vi "Read.vi"(8 "error in (no error)":errorcluster, 9 "Timeout (ms)":i32, 10 "Bytes to Read":i32, 11 "TCP Connection in":refnum<class "TCP Connection.lvclass">) -> (0 "error out":errorcluster, 1 "TimeOut?":bool, 2 "Data":string, 3 "TCP Connection out":refnum<class "TCP Connection.lvclass">)   [LabVIEW 2020, in "TCP Connection.lvclass"]
uses:
  <vilib>/gpm_packages/@cs/Network-interface/Source/TCP Interface/TCP Connection/TCP Connection.lvclass
  <vilib>/gpm_packages/@cs/Network-interface/Source/TCP Interface/TCP Connection/TCP Connection.lvclass/TCP Connection.ctl
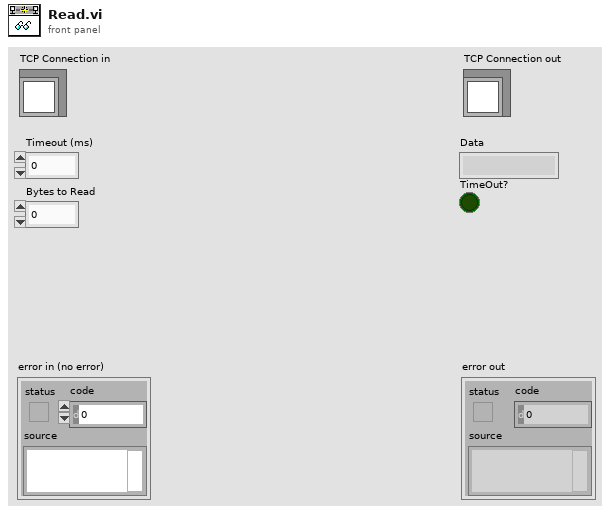
[diagram p1: front panel]
types:
  T1 = enum16{"Standard", "Buffered", "CRLF", "Immediate"}
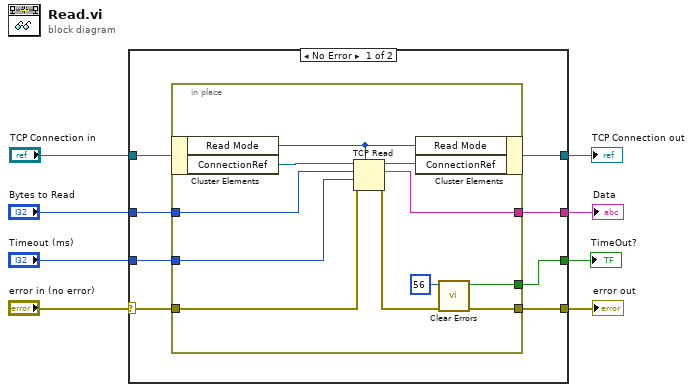
[diagram p0: block diagram]
diagram:
  n1 = case shown="No Error" "error in (no error)" {
    selector: "error in (no error)" -> [w15 w28]
    tunnel: "TCP Connection in" -> [w16 w29]
    tunnel: "Timeout (ms)" -> [w14 _]
    tunnel: "Bytes to Read" -> [w13 _]
    tunnel: [w12 w28] -> w4
    tunnel: [w11 _] -> w3
    tunnel: [w10 _] -> w2
    tunnel: [w9 w29] -> w1
    frame No Error {
      n2 = in-place {
        in-place-border: w15 -> [w25]
        in-place-border: w14 -> [w24]
        in-place-border: w13 -> [w23]
        in-place-border: [w21] -> w12
        in-place-border: [w19] -> w11
        in-place-border: [w18] -> w10
        n3 = in-place-cluster #1(w16) -> ("Read Mode"=w17:T1, "ConnectionRef"=w27:refnum<k5>)
        n4 = TCP Read(connection ID=w27, bytes to read=w23, error in (no error)=w25, 7:w17, 9:w24) -> (connection ID out=w26:refnum<k5>, data out=w18:string, error out=w22:errorcluster)
        n5 = in-place-cluster #1("Read Mode"=w17, "ConnectionRef"=w26) -> (w9:refnum<class "TCP Connection.lvclass">)
        n6 = call <vilib>:"Clear Errors.vi"("error in (no error)"=w22, "specific error code to clear (0: all)"=56) -> ("error out"=w21:errorcluster, "specific error cleared?"=w19:bool)  [unwired: 4 in]
      }
    }
    frame Error {
    }
  }
  "error out" <- w4
  "TCP Connection out" <- w1
  "Data" <- w2
  "TimeOut?" <- w3
